vi "Set Window Top Focus.vi"(8 "error in":errorcluster, 11 "Window data":T1) -> (0 "error out":errorcluster)   [LabVIEW 2011]
uses:
  Summitek/Win32/WinUSER/Windows/window state.ctl
  Summitek/Win32/WinUSER/Windows/hWnd.ctl
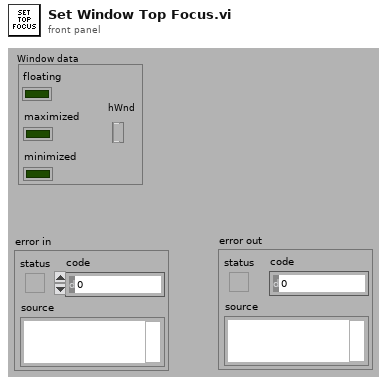
[diagram p1: front panel]
types:
  T1 = typedef "window state.ctl" = cluster{"minimized":bool, "maximized":bool, "floating":bool, "hWnd":T2}
  T2 = typedef "hWnd.ctl" = refnum<k1>
  T3 = enum32{"SW_SHOWDEFAULT", "SW_FORCEMINIMIZE", "SW_HIDE", "SW_MAXIMIZE", "SW_RESTORE", "SW_SHOW", "SW_SHOWMAXIMIZED", "SW_SHOWMINIMIZED", "SW_SHOWMINNOACTIVE", "SW_SHOWNA", "SW_SHOWNOACTIVATE", "SW_SHOWNORMAL"}
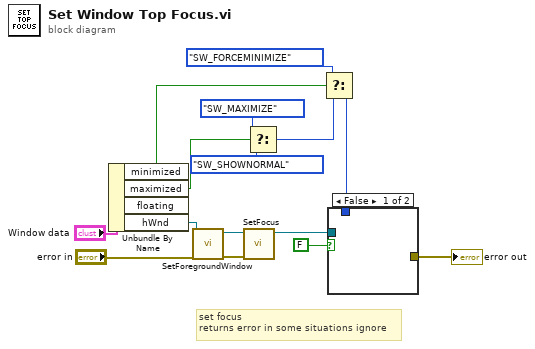
[diagram p0: block diagram]
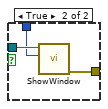
[diagram p2: hidden frame]
diagram:
  # "set focus \nreturns error in some situations ignore"
  n1 = Unbundle By Name("Window data") -> ("minimized"=w9:bool, "maximized"=w7:bool, "hWnd"=w11:T2)  [unwired: 1 out]
  n2 = call "SetForegroundWindow.vi"("error in (no error)"="error in", "hWnd (NULL)"=w11) -> ("error out"=w15:errorcluster, "dup hWnd"=w14:T2)  [unwired: 8 out]
  n3 = call "SetFocus.vi"("error in (no error)"=w15, "hWnd (NULL)"=w14) -> ("dup hWnd"=w10:T2)  [unwired: 9 out]
  n4 = Select(t=T3."SW_MAXIMIZE" ("nCmdShow\n(SW_SHOWNORMAL)"), s=w7, f=T3."SW_SHOWNORMAL" ("nCmdShow\n(SW_SHOWNORMAL)")) -> (s? t:f=w4:T3)
  n5 = Select(t=T3."SW_FORCEMINIMIZE" ("nCmdShow\n(SW_SHOWNORMAL)"), s=w9, f=w4) -> (s? t:f=w3:T3)
  n6 = case shown="False" FALSE {
    tunnel: w10 -> [_ w18]
    tunnel: w3 -> [_ w17]
    tunnel: [_ w16] -> w2
    frame False {
    }
    frame True {
      n7 = call "ShowWindow.vi"("nCmdShow\n(SW_SHOWNORMAL)"=w17, "hWnd (NULL)"=w18) -> ("error out"=w16:errorcluster)  [unwired: 1 in, 8 out]
    }
  }
  "error out" <- w2
